vi "WSVCAP SHL FPGA LL I2C Write CLK.vi"(0 "Bit In":bool, 11 "error in (no error)":errorcluster, 12 "UUT Set (0/1 (Legacy)":u8, 14 "Socket Mask":u64 format="%08x") -> (15 "error out":errorcluster)   [LabVIEW 2017]
uses:
  <vilib>/rvi/eio/common/nirviEmuTemplateMethod_errors.vi
  <vilib>/eio/EIONode/EIONode.xnode
  WSVCAP SHL FPGA LL I2C Debug Global.vi
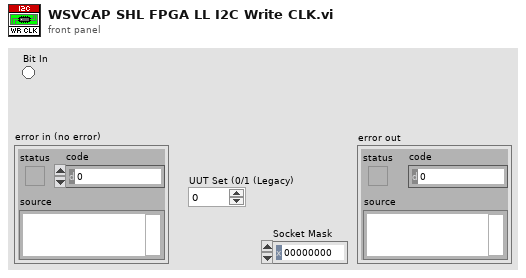
[diagram p1: front panel]
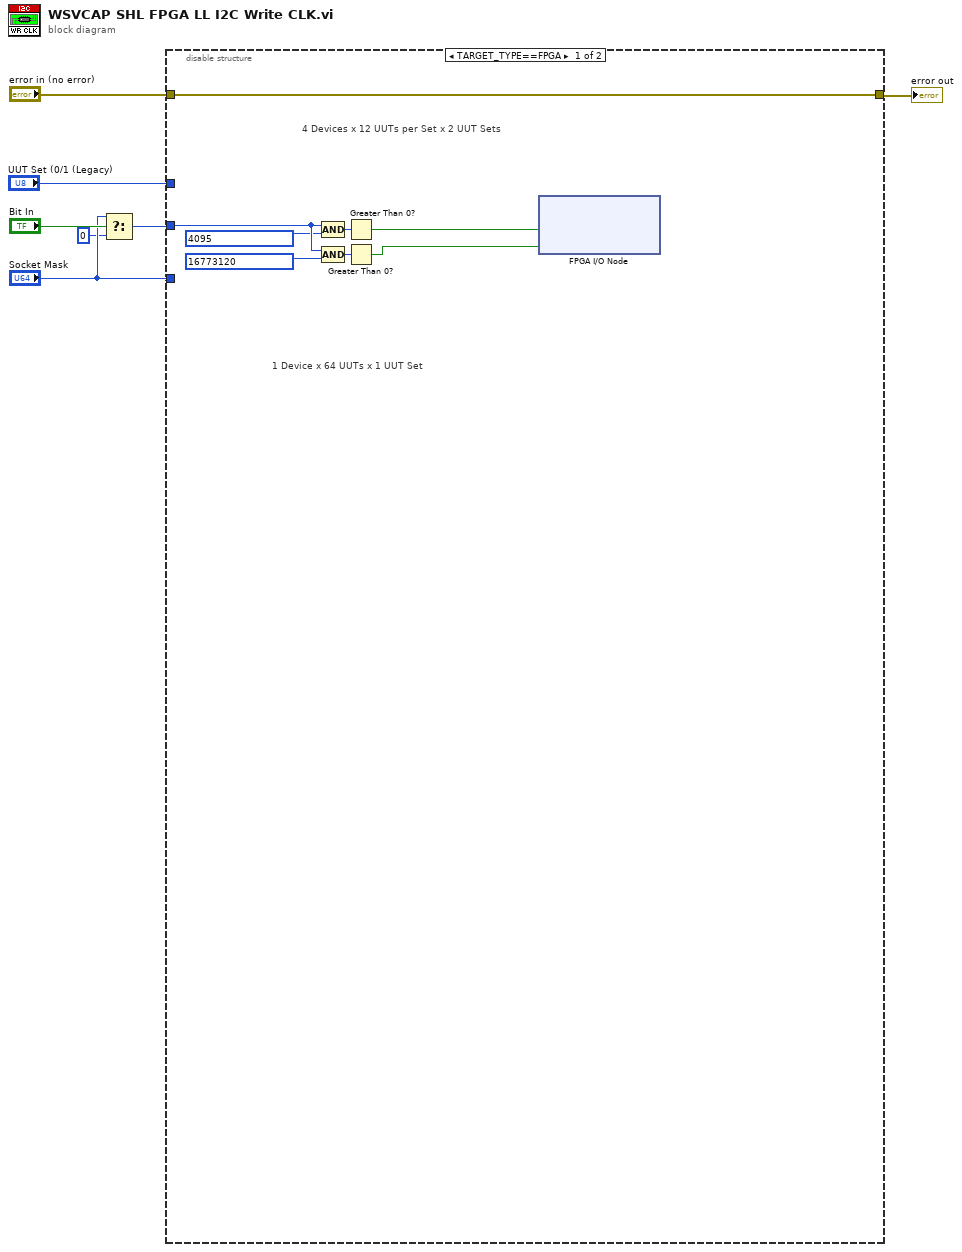
[diagram p0: block diagram]
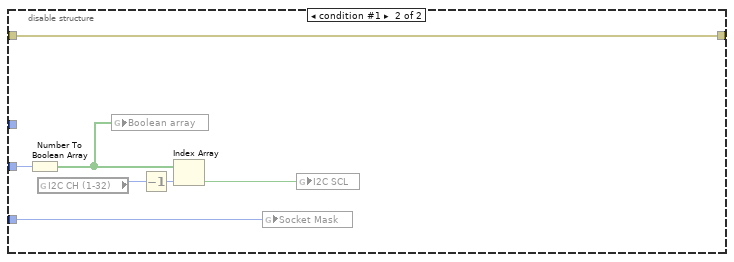
[diagram p2: hidden frame]
diagram:
  n1 = Select(t="Socket Mask", s="Bit In", f=u64 0) -> (s? t:f=w1:u64)
  n2 = disable-structure shown="TARGET_TYPE==FPGA" {
    disable-tunnel: w1 -> [w15 w18]
    disable-tunnel: [w14 w22] -> w7
    disable-tunnel: "error in (no error)" -> [w14 w22]
    disable-tunnel: "Socket Mask" -> [_ w16]
    disable-tunnel: "UUT Set (0/1 (Legacy)" -> [_ _]
    frame condition #0 (active) {
      # "1 Device x 64 UUTs x 1 UUT Set"
      # "4 Devices x 12 UUTs per Set x 2 UUT Sets"
      n3 = Compound Arithmetic op=AND(w15, u64 4095) -> (w13:u64)
      n4 = Compound Arithmetic op=AND(w15, u64 16773120) -> (w12:u64)
      n5 = Greater Than 0?(x=w13) -> (x > 0?=w11:bool)
      n6 = Greater Than 0?(x=w12) -> (x > 0?=w10:bool)
      n7 = xnode "FPGA I/O Node"("I2C_SCL_S1-12"=w11, "I2C_SCL_S13-24"=w10) -> ()  [unwired: 3 in, 3 out]
    }
    frame condition #1 {
      n8 = Number To Boolean Array(number=w18) -> (Boolean array=w17:bool[])
      n9 = global read "WSVCAP SHL FPGA LL I2C Debug Global.vi" "I2C CH (1-32)"() -> (w20:i32)
      n10 = global write "WSVCAP SHL FPGA LL I2C Debug Global.vi" "Boolean array"(w17) -> ()
      n11 = Decrement(x=w20) -> (x-1=w19:i32)
      n12 = Index Array(array=w17, index=w19) -> (element=w21:bool)
      n13 = global write "WSVCAP SHL FPGA LL I2C Debug Global.vi" "Socket Mask"(w16) -> ()
      n14 = global write "WSVCAP SHL FPGA LL I2C Debug Global.vi" "I2C SCL"(w21) -> ()
    }
  }
  "error out" <- w7
